vi "WSVCAP SHL Host LL RFFE Convert Channel Bytes to Bit Array.vi"(0 "RFFE Data [DUT Ordered]":u8[][](array[numeric]) format="%02x", 7 "Cycle CMD Lengths Out (bits)":u8[](array[numeric]), 9 "Cycle CMD Delay Out (ticks)":u32[](array[numeric])) -> (4 "Write Data":u64[](array[numeric]) format="%08x")   [LabVIEW 2012]
panel:
  # "0"
  # "7"
  # "0"
  # "1"
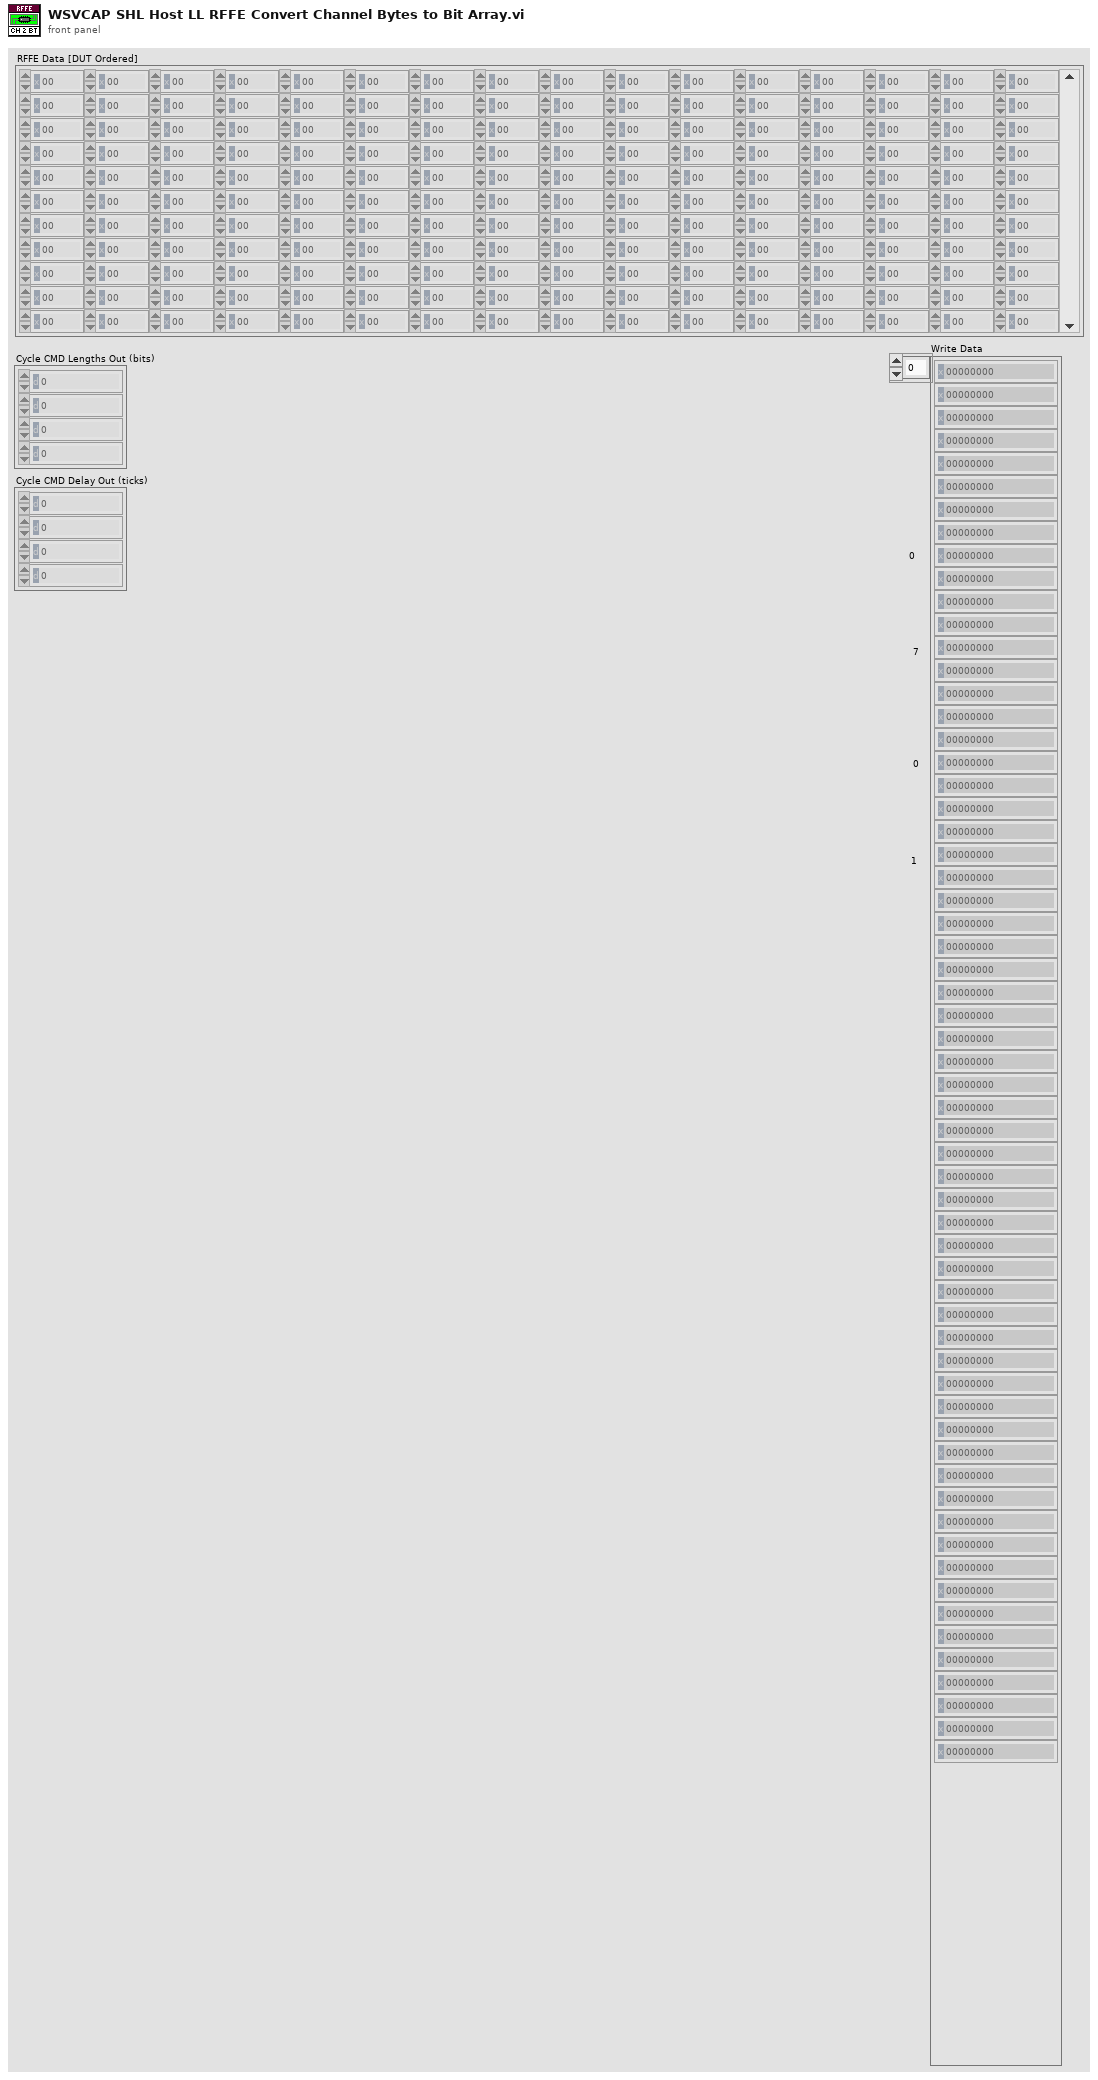
[diagram p1: front panel]
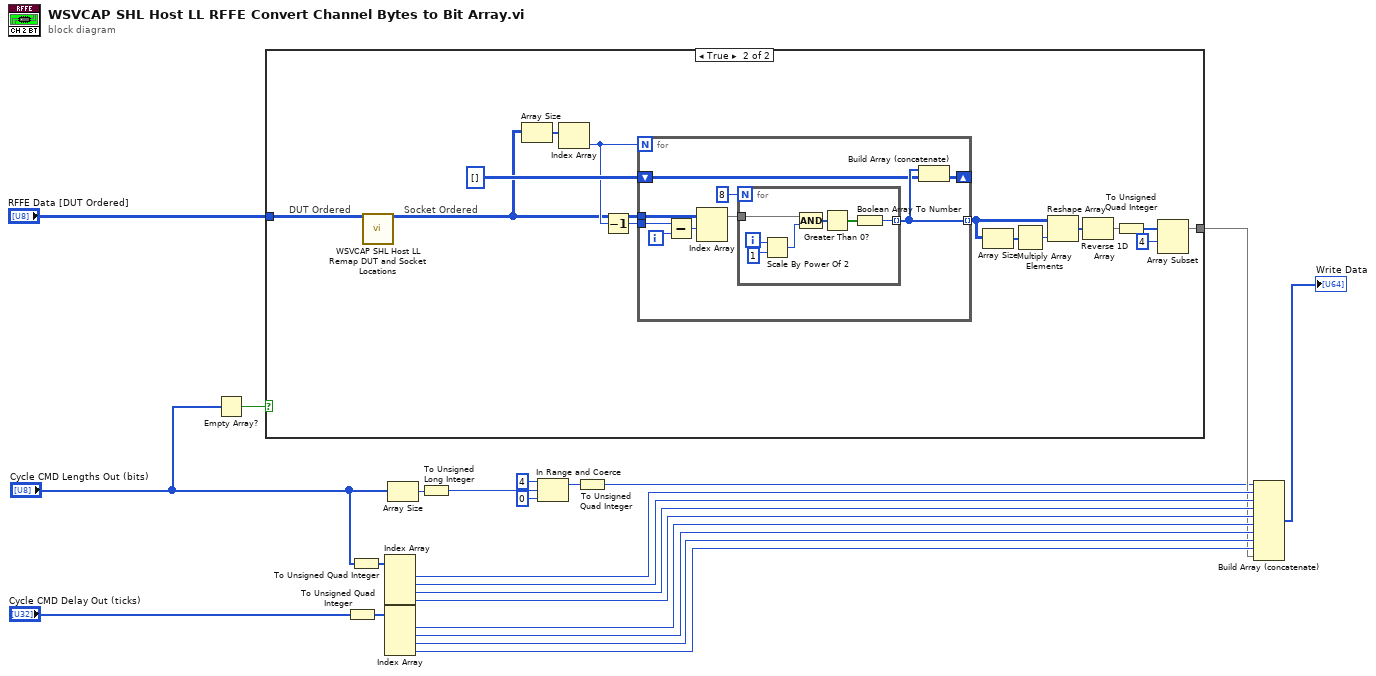
[diagram p0: block diagram]
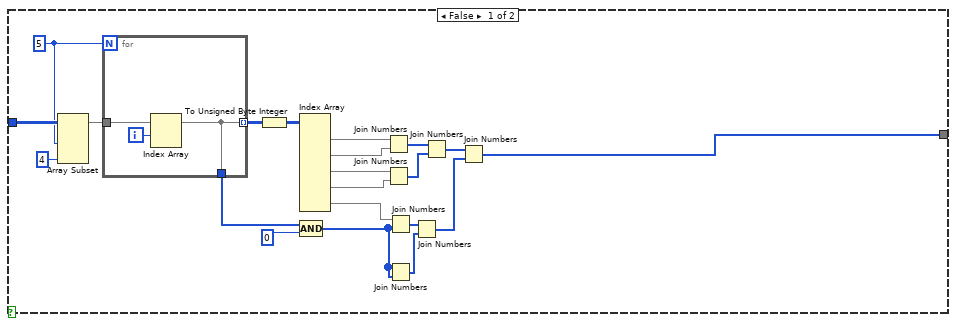
[diagram p2: hidden frame]
diagram:
  n1 = Empty Array?(array="Cycle CMD Lengths Out (bits)") -> (empty?=w3:bool)
  n2 = case shown="True" w3 {
    tunnel: "RFFE Data [DUT Ordered]" -> [w29 w51]
    tunnel: [w36 w48] -> w5
    frame False {
      w27 = 5
      n3 = Array Subset(array=w29, length (row)=w27, length (col)=4 ("length")) -> (w28:u8[][])  [unwired: 2 in]
      n4 = for {
        N: w27 -> [_]
        tunnel: w28 -> [w46]
        tunnel: [w44] -> w30 mode=indexing
        tunnel: [w44] -> w25
        i -> [w45]
        n5 = Index Array(array=w46, index (row)=w45) -> (element=w44:u8[])  [unwired: 1 in]
      }
      n6 = To Unsigned Byte Integer(number=w30) -> (unsigned 8bit integer=w35:u8[][])
      n7 = Index Array(array=w35) -> (element #1=w43:u8[], element #2=w42:u8[], element #3=w41:u8[], element #4=w40:u8[], element #5=w34:u8[])  [unwired: 10 in]
      n8 = Compound Arithmetic op=AND(w25, u8 0 ("Read Data")) -> (w24:u8[])
      n9 = Join Numbers(hi=w43, lo=w42) -> ((hi.lo)=w39:u16[])
      n10 = Join Numbers(hi=w41, lo=w40) -> ((hi.lo)=w38:u16[])
      n11 = Join Numbers(hi=w34, lo=w24) -> ((hi.lo)=w33:u16[])
      n12 = Join Numbers(hi=w24, lo=w24) -> ((hi.lo)=w32:u16[])
      n13 = Join Numbers(hi=w33, lo=w32) -> ((hi.lo)=w31:u32[])
      n14 = Join Numbers(hi=w39, lo=w38) -> ((hi.lo)=w37:u32[])
      n15 = Join Numbers(hi=w37, lo=w31) -> ((hi.lo)=w36:u64[])
    }
    frame True {
      # "Socket Ordered"
      # "DUT Ordered"
      n16 = call "WSVCAP SHL Host LL Remap DUT and Socket Locations.vi"("C1 DUT Ordered Data In"=w51) -> ("C1 Socket Ordered Data Out"=w50:u8[][])  [unwired: 13 in, 5 out]
      n17 = Array Size(array=w50) -> (size(s)=w56:i32[])
      n18 = Index Array(array=w56) -> (element=w54:i32)  [unwired: 1 in]
      n19 = Decrement(x=w54) -> (x-1=w53:i32)
      n20 = for {
        N: w54 -> [_]
        tunnel: w50 -> [w65]
        tunnel: [w68] -> w60 mode=indexing
        shift-right: [w67] -> _
        shift-left: u32[][] [] -> [w66]
        tunnel: w53 -> [w61]
        i -> [w63]
        n21 = Subtract(x=w61, y=w63) -> (x-y=w62:i32)
        n22 = Index Array(array=w65, index (row)=w62) -> (element=w64:u8[])  [unwired: 1 in]
        n23 = for {
          N: 8 -> [_]
          tunnel: w64 -> [w72]
          tunnel: [w71] -> w68 mode=indexing
          i -> [w74]
          n24 = Scale By Power Of 2(n=w74, x=u8 1) -> (x*2^n=w75:u8)
          n25 = Compound Arithmetic op=AND(w72, w75) -> (w76:u8[])
          n26 = Greater Than 0?(x=w76) -> (x > 0?=w70:bool[])
          n27 = Boolean Array To Number(Boolean array=w70) -> (number=w71:u32)
        }
        n28 = Build Array (concatenate)(w68, w66) -> (w67:u32[][])
      }
      n29 = Array Size(array=w60) -> (size(s)=w59:i32[])
      n30 = Multiply Array Elements(1:w59) -> (0:w58:i32)
      n31 = Reshape Array(w60, w58) -> (w55:u32[])
      n32 = Reverse 1D Array(array=w55) -> (reversed array=w52:u32[])
      n33 = To Unsigned Quad Integer(1:w52) -> (0:w49:u64[])
      n34 = Array Subset(array=w49, index=4) -> (w48:u64[])  [unwired: 1 in]
    }
  }
  n35 = To Unsigned Quad Integer(1:"Cycle CMD Delay Out (ticks)") -> (0:w2:u64[])
  n36 = To Unsigned Quad Integer(1:"Cycle CMD Lengths Out (bits)") -> (0:w14:u64[])
  n37 = Index Array(array=w14) -> (element #1=w16:u64, element #2=w15:u64, element #3=w13:u64, element #4=w12:u64)  [unwired: 4 in]
  n38 = Index Array(array=w2) -> (element #1=w11:u64, element #2=w10:u64, element #3=w9:u64, element #4=w8:u64)  [unwired: 4 in]
  n39 = Array Size(array="Cycle CMD Lengths Out (bits)") -> (size(s)=w21:i32)
  n40 = To Unsigned Long Integer(number=w21) -> (unsigned 32bit integer=w6:u32)
  n41 = In Range and Coerce(upper limit=u32 4, x=w6, lower limit=u32 0) -> (coerced(x)=w18:u32)  [unwired: 1 out]
  n42 = To Unsigned Quad Integer(1:w18) -> (0:w1:u64)
  n43 = Build Array (concatenate)(w1, w16, w15, w13, w12, w11, w10, w9, w8, w5) -> (→"Write Data":u64[])
